vi "ixon setup FT acquisition 2 - SubVI.vi"(5 "Shutter":i32(ring) items=["Auto", "Stay Open", "Always Closed"], 6 "EM CCD Gain":u16(slide)=230 scale=0.01..255.0, 7 "Interactive?":bool=TRUE, 8 "error in (no error)":errorcluster, 9 "Exposure Time (sec)":sgl(slide)=0.1 scale=0.001..10.0 scale format="%#_1g", 10 "Readout Settings":T1={"Acquisition Mode"=enum."Frame Transfer Run till Abort", "Pixel Rate"=enum."EM CCD 5 Mhz 14 bits", "High Capacity?"=FALSE, "V Shift Speed (us/row)"=enum."0.4 (not reccommended)", "V Shift Amplitude"=enum."normal", "Preamp Gain"=enum."1.0", "Trigger Mode"=0} {"Trigger Mode" items=["Internal", "External"]}, 11 "Image Size":T3={"H Bin"=1, "V Bin"=1, "Left"=1, "Top"=1, "Right"=512, "Bottom"=512}) -> (0 "error out":errorcluster, 1 "Actual Image Height":i32, 2 "Actual Image Width":i32, 3 "Actual Exposure Time (sec)":sgl format="%.4f")   [LabVIEW 2014]
doc: "Programs the hardware settings into the Andor iXon camera and prepares it for acquisition. This VI is currently designed for use with the \"Frame Transfer Run till Abort\" acquisition mode; it has not been tested with other modes."
uses:
  ixon readout settings - SubVI.ctl
  andor acquisition mode.ctl
  lib/Andorlib/atmcd32d.dll
panel:
  in  "Cancel":bool
  in  "Program Camera":bool
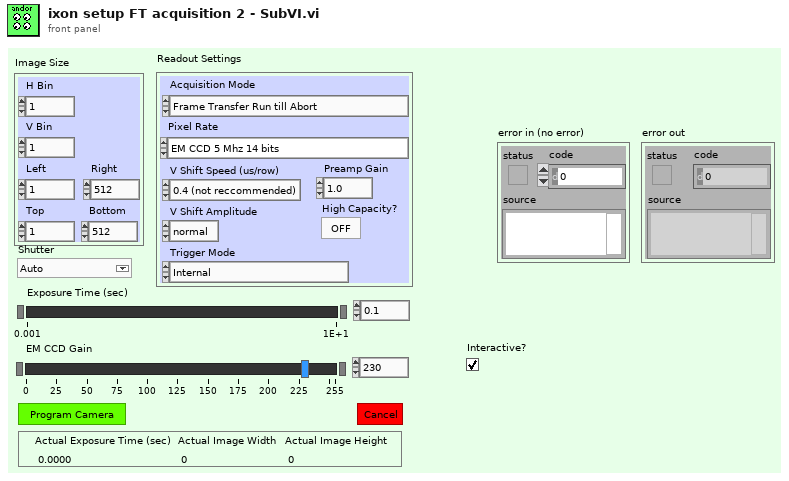
[diagram p1: front panel]
types:
  T1 = typedef "ixon readout settings - SubVI.ctl" = cluster{"Acquisition Mode":T2, "Pixel Rate":enum16{"EM CCD 10 Mhz 14 bits", "EM CCD 5 Mhz 14 bits", "EM CCD 3 Mhz 14 bits", "EM CCD 1 Mhz 16 bits", "Standard CCD 3 Mhz 14 bits", "Standard CCD 1 Mhz 16 bits"}, "High Capacity?":bool, "V Shift Speed (us/row)":enum16{"0.4 (not reccommended)", "0.6  (not reccommended)", "1.0  (not reccommended)", "1.8  (not reccommended)", "3.4  (not reccommended)", "6.6", "13.0"}, "V Shift Amplitude":enum16{"normal", "+1", "+2", "+3", "+4"}, "Preamp Gain":enum16{"1.0", "2.6"}, "Trigger Mode":u32}
  T2 = typedef "andor acquisition mode.ctl" = enum16{"(do not use)", "Single Scan", "Accumulate", "Kinetics", "Fast Kinetics", "Kinetics Run till Abort", "Frame Transfer", "Frame Transfer Run till Abort", "(do not use) ", "Time Delayed Integration"}
  T3 = cluster{"H Bin":i32, "V Bin":i32, "Left":i32, "Top":i32, "Right":i32, "Bottom":i32}
  T4 = cluster{"Adc Channel":i32, "H Shift Setting":i32, "EM on?":bool}[]
  T5 = enum16{"EM CCD 10 Mhz 14 bits", "EM CCD 5 Mhz 14 bits", "EM CCD 3 Mhz 14 bits", "EM CCD 1 Mhz 16 bits", "Standard CCD 3 Mhz 14 bits", "Standard CCD 1 Mhz 16 bits"}
  T6 = enum16{"0.4 (not reccommended)", "0.6  (not reccommended)", "1.0  (not reccommended)", "1.8  (not reccommended)", "3.4  (not reccommended)", "6.6", "13.0"}
  T7 = cluster{"Adc Channel":i32, "H Shift Setting":i32, "EM on?":bool}
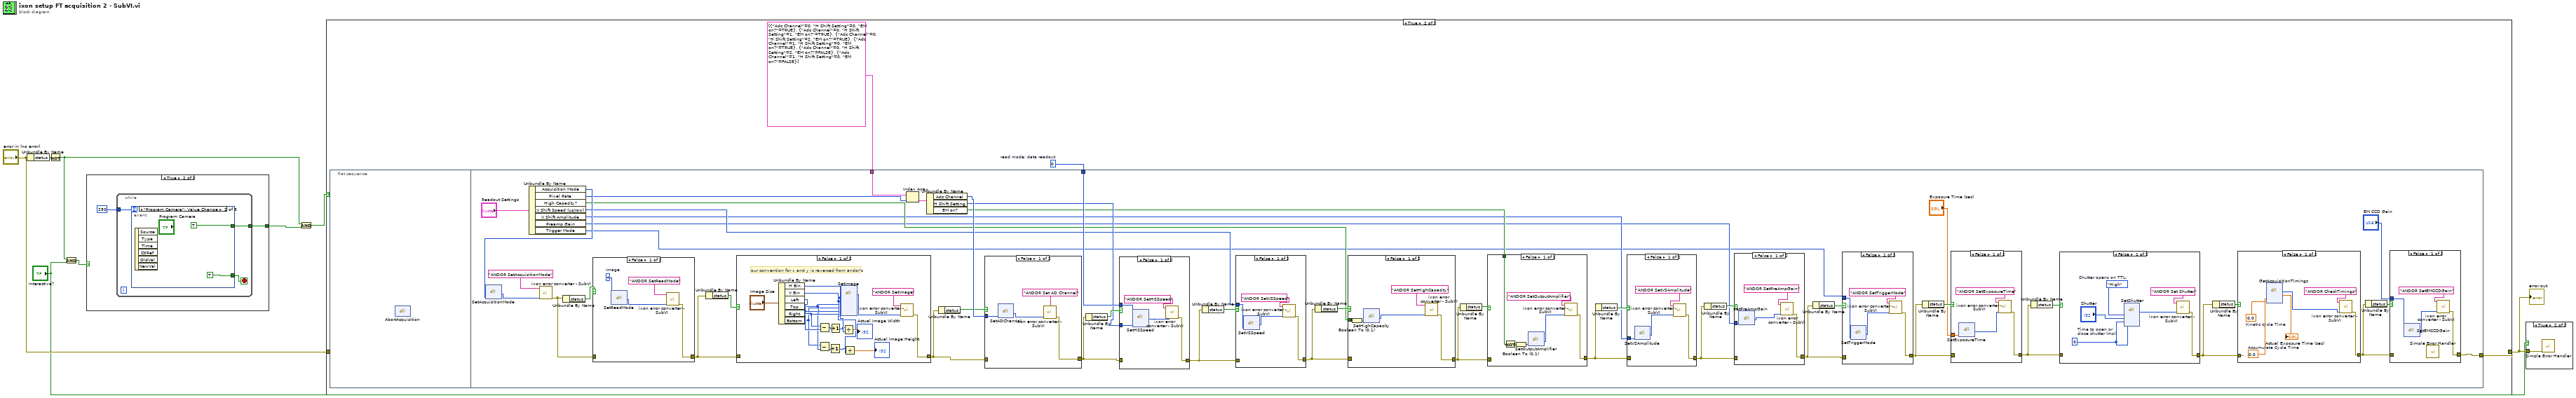
[diagram p0: block diagram]
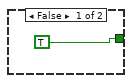
[diagram p3: hidden frame]
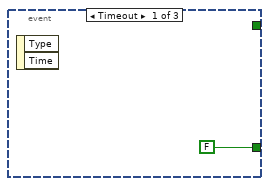
[diagram p4: hidden frame]
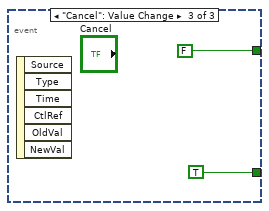
[diagram p5: hidden frame]
diagram:
  n1 = Unbundle By Name("error in (no error)") -> ("status"=w8:bool)
  n2 = Not(x=w8) -> (.not. x?=w4:bool)
  n3 = And(x=w4, y="Interactive?") -> (x .and. y?=w7:bool)
  n4 = case shown="True" w7 {
    tunnel: [TRUE w10] -> w6
    frame False {
    }
    frame True {
      n5 = while {
        tunnel: 250 -> [w14]
        tunnel: [w13] -> w10
        stop <- w12 stop-if-true
        n6 = event shown="[1] \"Program Camera\": Value Change" {
          selector: _ -> [_ _ _]
          dyn-events: _ -> [_ _ _]
          timeout: w14 -> [_ _ _]
          tunnel: [_ TRUE FALSE] -> w13
          tunnel: [FALSE TRUE TRUE] -> w12
          event Timeout {
            n7 = event-data() -> ()  [unwired: 3 out]
          }
          event "Program Camera": Value Change {
            n8 = event-data() -> ()  [unwired: 7 out]
          }
          event "Cancel": Value Change {
            n9 = event-data() -> ()  [unwired: 7 out]
          }
        }
      }
    }
  }
  n10 = And(x=w4, y=w6) -> (x .and. y?=w5:bool)
  n11 = case shown="True" w5 {
    tunnel: [w20 w21] -> w1
    tunnel: "error in (no error)" -> [w20 _]
    frame False {
    }
    frame True {
      w22 = 0  # read mode: data readout
      n12 = flat-sequence {
        tunnel: T4 [{"Adc Channel"=0, "H Shift Setting"=0, "EM on?"=TRUE}, {"Adc Channel"=0, "H Shift Setting"=1, "EM on?"=TRUE}, {"Adc Channel"=0, "H Shift Setting"=2, "EM on?"=TRUE}, {"Adc Channel"=1, "H Shift Setting"=0, "EM on?"=TRUE}, {"Adc Channel"=0, "H Shift Setting"=2, "EM on?"=FALSE}, {"Adc Channel"=1, "H Shift Setting"=0, "EM on?"=FALSE}] -> [w64]
        tunnel: w22 -> [w59]
        tunnel: [w24] -> w21
        frame #0 {
          n13 = dll-call lib="C:/Users/Bakir/Documents/Lambda2-Testing/lib/Andorlib/Atmcd32d.dll" fn="AbortAcquisition" label="Call Library Function\nAbort"() -> ()  [unwired: 3 in, 3 out]
        }
        frame #1 {
          n14 = Unbundle By Name("Readout Settings") -> ("Acquisition Mode"=w31:T2, "Pixel Rate"=w30:T5, "High Capacity?"=w28:bool, "V Shift Speed (us/row)"=w29:T6, "V Shift Amplitude"=w27:enum16{"normal", "+1", "+2", "+3", "+4"}, "Preamp Gain"=w26:enum16{"1.0", "2.6"}, "Trigger Mode"=w25:u32)
          n15 = dll-call lib="C:/Users/Bakir/Documents/Lambda2-Testing/lib/Andorlib/ATMCD32D.DLL" fn="SetAcquisitionMode"(w31) -> ("return type"=w70:u32)  [unwired: 3 in, 3 out]
          n16 = call "ixon error converter - SubVI.vi"("Andor error code"=w70, "source"="ANDOR SetAcquisitionMode") -> ("error out"=w67:errorcluster)  [unwired: 5 in]
          n17 = Unbundle By Name(w67) -> ("status"=w68:bool)
          n18 = case shown="False" w68 {
            tunnel: w67 -> [_ w160]
            tunnel: [w156 w160] -> w65
            frame False {
              w159 = u16 4  # Image
              n19 = dll-call lib="C:/Users/Bakir/Documents/Lambda2-Testing/lib/Andorlib/Atmcd32d.dll" fn="SetReadMode"(w159) -> (w157:u32)  [unwired: 3 in, 3 out]
              n20 = call "ixon error converter - SubVI.vi"("Andor error code"=w157, "source"="ANDOR SetReadMode") -> ("error out"=w156:errorcluster)  [unwired: 5 out]
            }
            frame True {
            }
          }
          n21 = Unbundle By Name(w65) -> ("status"=w66:bool)
          n22 = case shown="False" w66 {
            tunnel: w65 -> [_ w155]
            tunnel: [w152 w155] -> w60
            frame False {
              # "our convention for x and y is reversed from andor's"
              n23 = Unbundle By Name("Image Size") -> ("H Bin"=w148:i32, "V Bin"=w146:i32, "Left"=w141:i32, "Top"=w140:i32, "Right"=w142:i32, "Bottom"=w139:i32)
              n24 = Subtract(x=w142, y=w141) -> (x-y=w149:i32)
              n25 = Subtract(x=w139, y=w140) -> (x-y=w147:i32)
              n26 = Increment(x=w147) -> (x+1=w143:i32)
              n27 = Increment(x=w149) -> (x+1=w144:i32)
              n28 = dll-call lib="C:/Users/Bakir/Documents/Lambda2-Testing/lib/Andorlib/Atmcd32d.dll" fn="SetImage"(w148, w146, w140, w139, w141, w142) -> (w153:u32)  [unwired: 9 in, 2 out]
              n29 = Divide(x=w144, y=w148) -> (x/y=→"Actual Image Width":dbl)
              n30 = Divide(x=w143, y=w146) -> (x/y=→"Actual Image Height":dbl)
              n31 = call "ixon error converter - SubVI.vi"("Andor error code"=w153, "source"="ANDOR SetImage") -> ("error out"=w152:errorcluster)  [unwired: 5 in]
            }
            frame True {
            }
          }
          n32 = Index Array(array=w64, index=w30) -> (element=w63:T7)
          n33 = Unbundle By Name(w63) -> ("Adc Channel"=w62:i32, "H Shift Setting"=w56:i32, "EM on?"=w55:bool)
          n34 = Unbundle By Name(w60) -> ("status"=w61:bool)
          n35 = case shown="False" w61 {
            tunnel: w60 -> [_ w138]
            tunnel: w62 -> [w137 _]
            tunnel: [w134 w138] -> w57
            frame False {
              n36 = dll-call lib="C:/Users/Bakir/Documents/Lambda2-Testing/lib/Andorlib/Atmcd32d.dll" fn="SetADChannel" label="Set AD Channel"(w137) -> (w136:u32)  [unwired: 4 in, 2 out]
              n37 = call "ixon error converter - SubVI.vi"("Andor error code"=w136, "source"="ANDOR Set AD Channel") -> ("error out"=w134:errorcluster)  [unwired: 5 in]
            }
            frame True {
            }
          }
          n38 = Unbundle By Name(w57) -> ("status"=w58:bool)
          n39 = case shown="False" w58 {
            tunnel: [w130 w133] -> w52
            tunnel: w59 -> [w129 _]
            tunnel: w57 -> [_ w133]
            tunnel: w56 -> [w128 _]
            frame False {
              n40 = dll-call lib="C:/Users/Bakir/Documents/Lambda2-Testing/lib/Andorlib/Atmcd32d.dll" fn="SetHSSpeed"(w129, w128) -> (w132:u32)  [unwired: 5 in, 2 out]
              n41 = call "ixon error converter - SubVI.vi"("Andor error code"=w132, "source"="ANDOR SetHSSpeed") -> ("error out"=w130:errorcluster)  [unwired: 5 in]
            }
            frame True {
            }
          }
          n42 = Unbundle By Name(w52) -> ("status"=w53:bool)
          n43 = case shown="False" w53 {
            tunnel: [w125 w127] -> w51
            tunnel: w29 -> [w124 _]
            tunnel: w52 -> [_ w127]
            frame False {
              n44 = dll-call lib="C:/Users/Bakir/Documents/Lambda2-Testing/lib/Andorlib/Atmcd32d.dll" fn="SetVSSpeed"(w124) -> (w123:u32)  [unwired: 3 in, 3 out]
              n45 = call "ixon error converter - SubVI.vi"("Andor error code"=w123, "source"="ANDOR SetVSSpeed") -> ("error out"=w125:errorcluster)  [unwired: 5 in]
            }
            frame True {
            }
          }
          n46 = Unbundle By Name(w51) -> ("status"=w54:bool)
          n47 = case shown="False" w54 {
            tunnel: [w120 w122] -> w50
            tunnel: w28 -> [w118 _]
            tunnel: w51 -> [_ w122]
            frame False {
              n48 = Boolean To (0,1)(Boolean=w118) -> (0, 1=w119:i16)
              n49 = dll-call lib="C:/Users/Bakir/Documents/Lambda2-Testing/lib/Andorlib/Atmcd32d.dll" fn="SetHighCapacity"(w119) -> (w117:u32)  [unwired: 3 in, 3 out]
              n50 = call "ixon error converter - SubVI.vi"("Andor error code"=w117, "source"="ANDOR SetHighCapacity") -> ("error out"=w120:errorcluster)  [unwired: 5 in]
            }
            frame True {
            }
          }
          n51 = Unbundle By Name(w50) -> ("status"=w49:bool)
          n52 = case shown="False" w49 {
            tunnel: [w114 w116] -> w48
            tunnel: w55 -> [w111 _]
            tunnel: w50 -> [_ w116]
            frame False {
              n53 = Not(x=w111) -> (.not. x?=w112:bool)
              n54 = Boolean To (0,1)(Boolean=w112) -> (0, 1=w113:i16)
              n55 = dll-call lib="C:/Users/Bakir/Documents/Lambda2-Testing/lib/Andorlib/Atmcd32d.dll" fn="SetOutputAmplifier"(w113) -> (w110:u32)  [unwired: 3 in, 3 out]
              n56 = call "ixon error converter - SubVI.vi"("Andor error code"=w110, "source"="ANDOR SetOutputAmplifier") -> ("error out"=w114:errorcluster)  [unwired: 5 in]
            }
            frame True {
            }
          }
          n57 = Unbundle By Name(w48) -> ("status"=w47:bool)
          n58 = case shown="False" w47 {
            tunnel: [w107 w109] -> w46
            tunnel: w48 -> [_ w109]
            tunnel: w27 -> [w105 _]
            frame False {
              n59 = dll-call lib="C:/Users/Bakir/Documents/Lambda2-Testing/lib/Andorlib/Atmcd32d.dll" fn="SetVSAmplitude"(w105) -> (w106:u32)  [unwired: 3 in, 3 out]
              n60 = call "ixon error converter - SubVI.vi"("Andor error code"=w106, "source"="ANDOR SetVSAmplitude") -> ("error out"=w107:errorcluster)  [unwired: 5 in]
            }
            frame True {
            }
          }
          n61 = Unbundle By Name(w46) -> ("status"=w45:bool)
          n62 = case shown="False" w45 {
            tunnel: [w102 w104] -> w42
            tunnel: w46 -> [_ w104]
            tunnel: w26 -> [w100 _]
            frame False {
              n63 = dll-call lib="C:/Users/Bakir/Documents/Lambda2-Testing/lib/Andorlib/Atmcd32d.dll" fn="SetPreAmpGain"(w100) -> (w101:u32)  [unwired: 3 in, 3 out]
              n64 = call "ixon error converter - SubVI.vi"("Andor error code"=w101, "source"="ANDOR SetPreAmpGain") -> ("error out"=w102:errorcluster)  [unwired: 5 in]
            }
            frame True {
            }
          }
          n65 = Unbundle By Name(w42) -> ("status"=w41:bool)
          n66 = case shown="False" w41 {
            tunnel: [w97 w99] -> w43
            tunnel: w42 -> [_ w99]
            tunnel: w25 -> [w95 _]
            frame False {
              n67 = dll-call lib="C:/Users/Bakir/Documents/Lambda2-Testing/lib/Andorlib/Atmcd32d.dll" fn="SetTriggerMode"(w95) -> (w96:u32)  [unwired: 4 in, 2 out]
              n68 = call "ixon error converter - SubVI.vi"("Andor error code"=w96, "source"="ANDOR SetTriggerMode") -> ("error out"=w97:errorcluster)  [unwired: 5 in]
            }
            frame True {
            }
          }
          n69 = Unbundle By Name(w43) -> ("status"=w44:bool)
          n70 = case shown="False" w44 {
            tunnel: [w92 w94] -> w36
            tunnel: w43 -> [_ w94]
            tunnel: "Exposure Time (sec)" -> [w91 _]
            frame False {
              n71 = dll-call lib="C:/Users/Bakir/Documents/Lambda2-Testing/lib/Andorlib/Atmcd32d.dll" fn="SetExposureTime"(w91) -> (w90:u32)  [unwired: 4 in, 2 out]
              n72 = call "ixon error converter - SubVI.vi"("Andor error code"=w90, "source"="ANDOR SetExposureTime") -> ("error out"=w92:errorcluster)  [unwired: 5 in]
            }
            frame True {
            }
          }
          n73 = Unbundle By Name(w36) -> ("status"=w39:bool)
          n74 = case shown="False" w39 {
            tunnel: [w87 w89] -> w35
            tunnel: w36 -> [_ w89]
            frame False {
              w86 = 0  # Time to open or close shutter (ms):
              w85 = enum16{"Low", "High"}."High"  # Shutter opens on TTL:
              n75 = dll-call lib="C:/Users/Bakir/Documents/Lambda2-Testing/lib/Andorlib/Atmcd32d.dll" fn="SetShutter" label="Set Shutter"(w85, "Shutter", w86, w86) -> (w83:u32)  [unwired: 6 in, 3 out]
              n76 = call "ixon error converter - SubVI.vi"("Andor error code"=w83, "source"="ANDOR Set Shutter") -> ("error out"=w87:errorcluster)  [unwired: 5 in]
            }
            frame True {
            }
          }
          n77 = Unbundle By Name(w35) -> ("status"=w38:bool)
          n78 = case shown="False" w38 {
            tunnel: [w80 w82] -> w34
            tunnel: w35 -> [_ w82]
            frame False {
              w78 = sgl 0.0  # Accumulate Cycle Time
              w77 = sgl 0.0  # Kinetic cycle Time
              n79 = dll-call lib="C:/Users/Bakir/Documents/Lambda2-Testing/lib/Andorlib/Atmcd32d.dll" fn="GetAcquisitionTimings" label="CheckTimings"(w78, w77) -> (w76:u32, →"Actual Exposure Time (sec)":sgl)  [unwired: 3 in, 5 out]
              n80 = call "ixon error converter - SubVI.vi"("Andor error code"=w76, "source"="ANDOR CheckTimings") -> ("error out"=w80:errorcluster)  [unwired: 5 in]
            }
            frame True {
            }
          }
          n81 = Unbundle By Name(w34) -> ("status"=w37:bool)
          n82 = case shown="False" w37 {
            tunnel: [w73 w75] -> w24
            tunnel: w34 -> [_ w75]
            tunnel: "EM CCD Gain" -> [w71 _]
            frame False {
              n83 = dll-call lib="C:/Users/Bakir/Documents/Lambda2-Testing/lib/Andorlib/Atmcd32d.dll" fn="SetEMCCDGain"(w71) -> (w72:u32)  [unwired: 3 in, 3 out]
              n84 = call "ixon error converter - SubVI.vi"("Andor error code"=w72, "source"="ANDOR SetEMCCDGain") -> ("error out"=w73:errorcluster)  [unwired: 5 in]
            }
            frame True {
            }
          }
          n85 = call <vilib>:"Simple Error Handler.vi"() -> ()  [unwired: 2 in, 8 out]
        }
      }
    }
  }
  "error out" <- w1
  n86 = case shown="True" "Interactive?" {
    tunnel: w1 -> [_ w161]
    frame False {
    }
    frame True {
      n87 = call <vilib>:"Simple Error Handler.vi"("error in (no error)"=w161) -> ()  [unwired: 1 in, 8 out]
    }
  }
